vi "DAQmx Create Channel (CI-Semi Period).vi"(0 "task in":refnum<k21>, 1 "maximum value":dbl=0.1 format="%.6f", 2 "minimum value":dbl=1e-06 format="%.6f", 5 "counter":tag, 7 "name to assign":string, 9 "units":i32(ring)=10364 items=["Seconds"=10364, "Ticks"=10304, "From Custom Scale"=10065], 11 "error in":errorcluster, 12 "custom scale name":tag) -> (4 "task out":refnum<k21>, 15 "error out":errorcluster)   [LabVIEW 2013]
doc: "Creates a channel to measure the time between state transitions of a digital signal. With the exception of devices that support multi-counter tasks, you can create only one counter input channel at a time with this VI because a task can contain only one counter input channel. To read from multiple counters simultaneously, use a separate task for each counter. Connect the input signal to the default input terminal of the counter unless you select a different input terminal."
uses:
  <resource>/objmgr/daqmx.rc
panel:
  # "input limits"
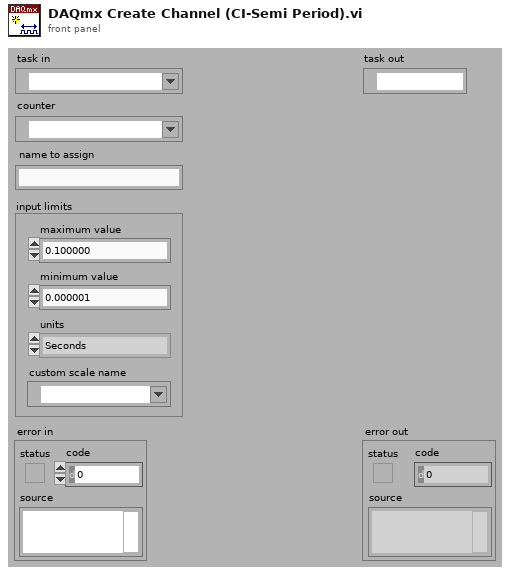
[diagram p1: front panel]
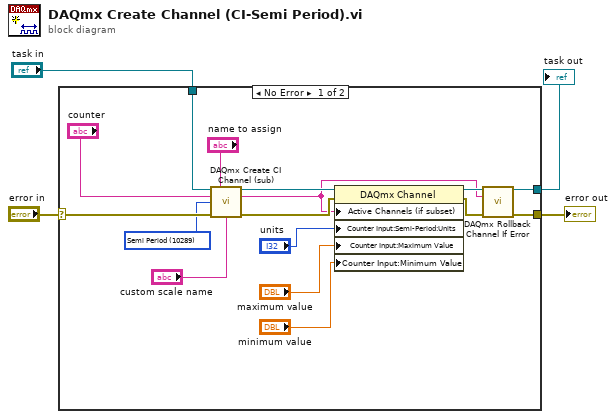
[diagram p0: block diagram]
diagram:
  n1 = case shown="No Error" "error in" {
    selector: "error in" -> [w19 w21]
    tunnel: "task in" -> [w20 w22]
    tunnel: [w8 w22] -> w2
    tunnel: [w7 w21] -> w1
    frame No Error {
      w14 = 10289 items=["Count Events"=10125, "Frequency"=10179, "Period"=10256, "Pulse width"=10267, "Semi Period"=10289] ("measurement type")
      n2 = call "DAQmx Create CI Channel (sub).vi"("task in"=w20, "virtual channel name"="name to assign", "physical channel name"="counter", "measurement type"=w14, "error in"=w19, "custom scale"="custom scale name") -> ("task out"=w12:refnum<k21>, "channel names"=w5:string, "error out"=w17:errorcluster)  [unwired: 7 out]
      n3 = property class="DAQmx Channel"(reference=w12, error in=w17, "Active Channels (if subset)"=w5, "Counter Input:Semi-Period:Units"="units", "Counter Input:Maximum Value"="maximum value", "Counter Input:Minimum Value"="minimum value") -> (reference out=w9:refnum<k21>, error out=w6:errorcluster)
      n4 = call "DAQmx Rollback Channel If Error.vi"("task in"=w9, "channel names"=w5, "error in"=w6) -> ("task out"=w8:refnum<k21>, "error out"=w7:errorcluster)  [unwired: 11 out]
    }
    frame Error {
    }
  }
  "error out" <- w1
  "task out" <- w2
